vi "ClearAllSelections.vi"(1 "old Table":string[][](array[string])) -> (0 "New Table":string[][](array[string]))   [LabVIEW 2014]
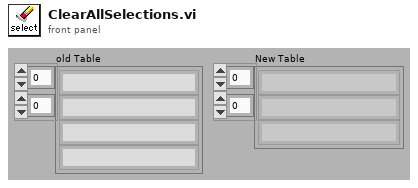
[diagram p1: front panel]
types:
  T1 = typedef "ParamterCluster.ctl" = cluster{"bounce?":bool, "black?":bool, "slide number":i32, "hide?":bool, "selection":bool}
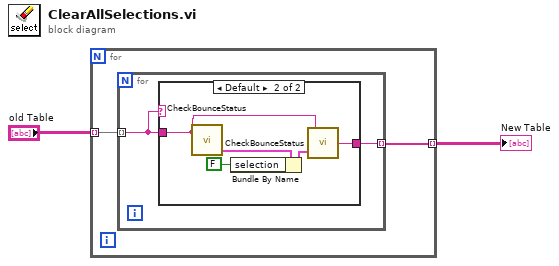
[diagram p0: block diagram]
diagram:
  n1 = for {
    tunnel: "old Table" -> [w4] mode=indexing
    tunnel: [w3] -> w2 mode=indexing
    n2 = for {
      tunnel: w4 -> [w5] mode=indexing
      tunnel: [w6] -> w3 mode=indexing
      n3 = case shown="Default" w5 {
        tunnel: w5 -> [w7 w9]
        tunnel: [w7 w8] -> w6
        frame "" {
        }
        frame Default {
          n4 = call "CheckBounceStatus.vi"("File Name"=w9) -> ("Parameters"=w10:T1)  [unwired: 1 in, 2 out]
          n5 = Bundle By Name(cluster=w10, "selection"=FALSE) -> (w12:T1)
          n6 = call "CheckBounceStatus.vi"("Parameters in"=w12, "File Name"=w9) -> ("With parameters"=w8:string)  [unwired: 2 out]
        }
      }
    }
  }
  "New Table" <- w2
